vi "matrix_mult.vi"(10 "Weights":dbl[][](array[numeric]), 11 "Input Array":dbl[](array[numeric])) -> (3 "Matrix Product":dbl[](array[numeric]))   [LabVIEW 2018]
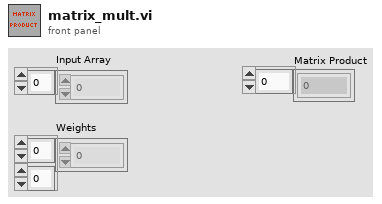
[diagram p1: front panel]
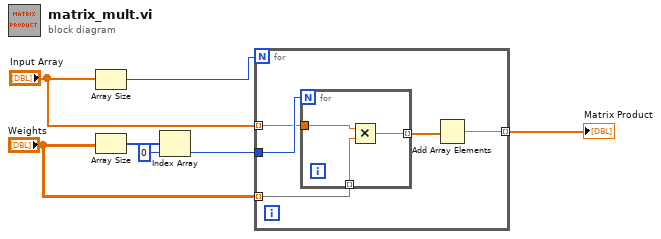
[diagram p0: block diagram]
diagram:
  n1 = Array Size(array="Input Array") -> (size(s)=w5:i32)
  n2 = Array Size(array="Weights") -> (size(s)=w7:i32[])
  n3 = Index Array(array=w7, index=0) -> (element=w4:i32)
  n4 = for {
    N: w5 -> [_]
    tunnel: w4 -> [w12]
    tunnel: "Input Array" -> [w11] mode=indexing
    tunnel: "Weights" -> [w10] mode=indexing
    tunnel: [w8] -> w1 mode=indexing
    n5 = for {
      N: w12 -> [_]
      tunnel: w11 -> [w15]
      tunnel: w10 -> [w14] mode=indexing
      tunnel: [w13] -> w9 mode=indexing
      n6 = Multiply(x=w15, y=w14) -> (x*y=w13:dbl)
    }
    n7 = Add Array Elements(numeric array=w9) -> (sum=w8:dbl)
  }
  "Matrix Product" <- w1
